vi "Close & Save Project.vi"(8 "error in (no error)":errorcluster, 9 "Project in":refnum<vi>) -> (0 "error out":errorcluster, 2 "Path":path)   [LabVIEW 2018]
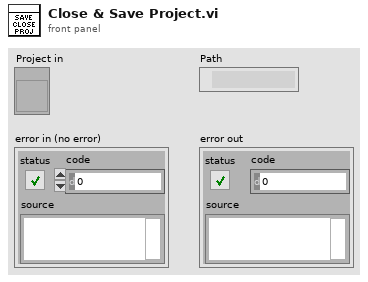
[diagram p1: front panel]
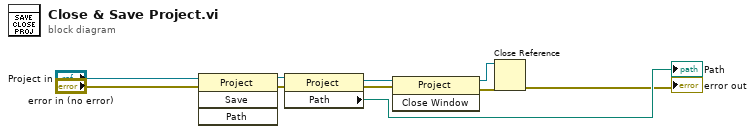
[diagram p0: block diagram]
diagram:
  n1 = invoke class="Project" method="Save"(reference="Project in", error in="error in (no error)") -> (reference out=w5:refnum<vi>, error out=w4:errorcluster)  [unwired: 2 in, 2 out]
  n2 = property class="Project"(reference=w5, error in=w4) -> (reference out=w7:refnum<vi>, error out=w6:errorcluster, "Path"=→"Path":path)
  n3 = invoke class="Project" method="Close Window"(reference=w7, error in=w6) -> (reference out=w2:refnum<vi>, error out=w1:errorcluster)  [unwired: 1 in, 1 out]
  n4 = Close Reference(reference=w2, error in (no error)=w1) -> (error out=→"error out":errorcluster)
